vi "Periodic Tasks.vi"(8 "error in":errorcluster) -> ()   [LabVIEW 2014]
doc: "This VI runs in parallel to other tasks. It can contain as many user-defined periodic loops as you need. These can carry out PID or other sorts of timed response."
uses:
  <vilib>/Rock Robotics/WPI/Solenoid/WPI_SolenoidValue.ctl
  <vilib>/Rock Robotics/WPI/Joystick/WPI_JoystickGetSetRefNum.vi
  <vilib>/Rock Robotics/WPI/RobotDrive/WPI_RobotDriveGetSetRefNum.vi
  Robot Global Data.vi
  <vilib>/Rock Robotics/WPI/Solenoid/WPI_SolenoidSetEnum.vi
panel:
  out "Encoder (INCH)":dbl format="%#_10g"
  in  "error in 2":errorcluster
  in  "X-Slew Rate":dbl=0.05
  in  "Y-Slew Rate":dbl=0.05
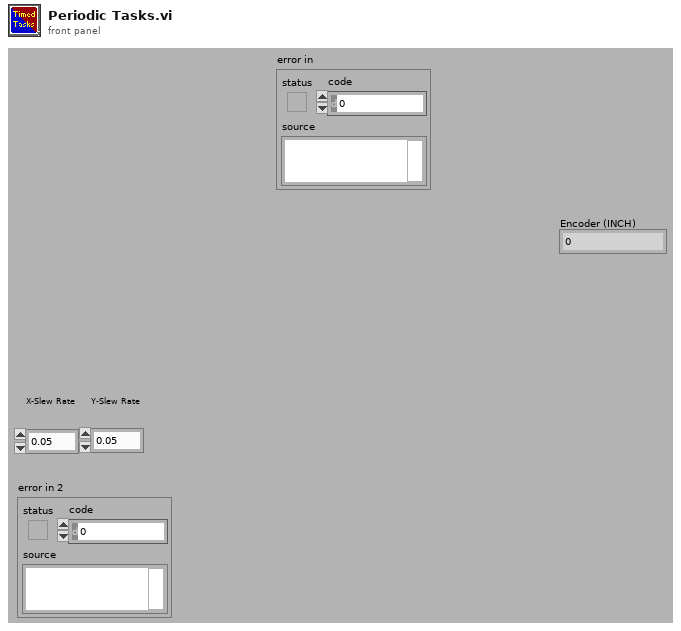
[diagram p1: front panel]
types:
  T1 = typedef "WPI_EncoderDevRef.ctl" = cluster{"DevStatus":errorcluster, "EncoderIndex":T2, "CounterIndex":T3, "DistancePerCount":dbl, "Decoding Type":T4}
  T2 = typedef "FPGA_EncoderIdx.ctl" = enum8{"Enc 0", "Enc 1", "Enc 2", "Enc 3", "Enc 4", "Enc 5", "Enc 6", "Enc 7", "Invalid"}
  T3 = typedef "FPGA_CounterCtrSystemIndex.ctl" = enum8{"Ctr 0", "Ctr 1", "Ctr 2", "Ctr 3", "Ctr 4", "Ctr 5", "Ctr 6", "Ctr 7", "Invalid"}
  T4 = typedef "WPI_EncoderType.ctl" = enum16{"1x", "2x", "4x"}
  T5 = typedef "WPI_RobotDriveDevRef.ctl" = cluster{"DevStatus":errorcluster, "Motors[]":T6[], "Square Inputs":bool, "Max Output":dbl}
  T6 = typedef "WPI_MotorControlDeviceRef.ctl" = cluster{"DeviceStatus":errorcluster, "Type":T7, "PWM":cluster{"Controller":T8, "PWM Channel":T9, "DeadBand":T10}, "CAN":cluster{"Device Number":u8, "Control Mode":T11, "Semaphore":T12, "Max Vout":dbl, "TalonSRX Control Mode":T13}, "Invert":bool, "TransformRef":T14, "InvTransformRef":T14}
  T7 = typedef "WPI_MotorControlType.ctl" = enum16{"PWM", "CAN", "CANTalonSRX"}
  T8 = typedef "FPGA_TypedefDigitalModule.ctl" = enum16{"Controller 1"}
  T9 = typedef "FPGA_DIOPWMChannel.ctl" = enum8{"PWM 0", "PWM 1", "PWM 2", "PWM 3", "PWM 4", "PWM 5", "PWM 6", "PWM 7", "PWM 8", "PWM 9", "PWM MXP 0", "PWM MXP 1", "PWM MXP 2", "PWM MXP 3", "PWM MXP 4", "PWM MXP 5", "PWM MXP 6", "PWM MXP 7", "PWM MXP 8", "PWM MXP 9", "Invalid"}
  T10 = typedef "WPI_PWMDeadband.ctl" = cluster{"Name":string, "maxPositivePwm":i32, "minPositivePwm":i32, "centerPwm":i32, "maxNegativePwm":i32, "minNegativePwm":i32, "angularRange":u16}
  T11 = typedef "WPI_CANJaguar_ControlMode.ctl" = enum8{"Percent VBus", "Current", "Speed", "Position", "Voltage"}
  T12 = typedef "Semaphore RefNum" = refnum<k1>
  T13 = typedef "WPI_CANTalonSRX_APIControlMode.ctl" = enum8{"Percent VBus", "Speed", "Position", "Slave", "Unchanged / Invalid"}
  T14 = typedef "WPI_PWMTransform_ConPane.ctl" = refnum<vi>
  T15 = typedef "WPI_JoystickDevRef.ctl" = cluster{"Device":T16}
  T16 = typedef "WPI_JoystickDeviceEnum.ctl" = enum16{"USB 0", "USB 1", "USB 2", "USB 3", "USB 4", "USB 5"}
  T17 = cluster{"JoystickDevRef":T15, "RobotDriveDevRef":T5}
  T18 = typedef "WPI_SolenoidDevRef.ctl" = cluster{"DevStatus":errorcluster, "Pneumatics Control Module":u8, "Forward Solenoid Channel":T19, "Reverse Solenoid Channel":T19}
  T19 = typedef "WPI_SolenoidChannel.ctl" = enum8{"Solenoid 0", "Solenoid 1", "Solenoid 2", "Solenoid 3", "Solenoid 4", "Solenoid 5", "Solenoid 6", "Solenoid 7", "Invalid"}
  T20 = typedef "WPI_SolenoidValue.ctl" = enum16{"Off", "On", "Forward", "Reverse"}
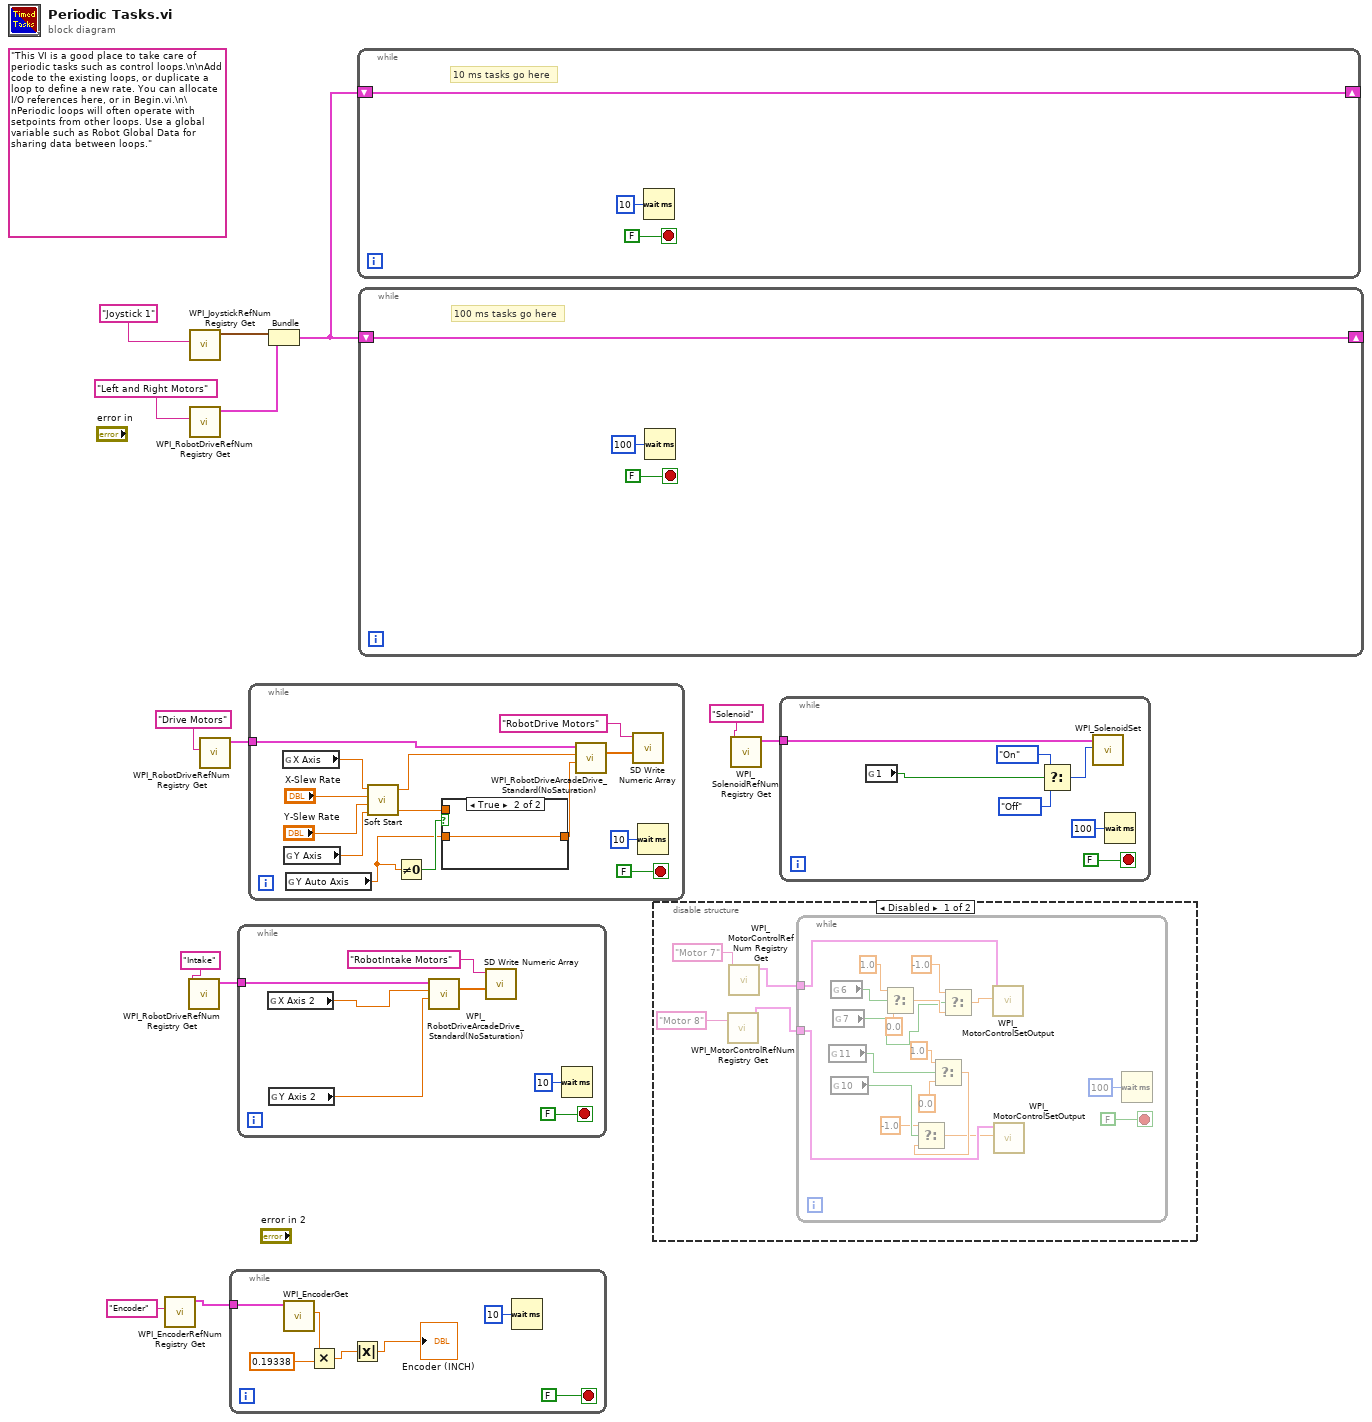
[diagram p0: block diagram]
diagram:
  (unwired) "This VI is a good place to take care of periodic tasks such as control loops.\n\nAdd code to the existing loops, or duplicate a loop to define a new rate. You can allocate I/O references here, or in Begin.vi.\n\nPeriodic loops will often operate with setpoints from other loops. Use a global variable such as Robot Global Data for sharing data between loops."
  n1 = call <vilib>:"WPI_EncoderRefNum Registry Get.vi"("refnum name"="Encoder") -> ("EncoderDevRef"=w1:T1)  [unwired: 9 in, 1 out]
  n2 = call <vilib>:"WPI_RobotDriveRefNum Registry Get.vi"("refnum name"="Intake") -> ("RobotDriveDevRef"=w3:T5)  [unwired: 1 in, 9 out]
  n3 = call <vilib>:"WPI_JoystickRefNum Registry Get.vi"("refnum name"="Joystick 1") -> ("JoystickDevRef"=w11:T15)  [unwired: 1 in, 9 out]
  n4 = call <vilib>:"WPI_RobotDriveRefNum Registry Get.vi"("refnum name"="Left and Right Motors") -> ("RobotDriveDevRef"=w10:T5)  [unwired: 1 in, 9 out]
  n5 = call <vilib>:"WPI_RobotDriveRefNum Registry Get.vi"("refnum name"="Drive Motors") -> ("RobotDriveDevRef"=w7:T5)  [unwired: 1 in, 9 out]
  n6 = while {
    tunnel: w1 -> [w19]
    stop <- FALSE stop-if-true
    n7 = call <vilib>:"WPI_EncoderGet.vi"("EncoderDevRef"=w19) -> ("Distance"=w18:dbl)  [unwired: 5 in, 5 out]
    n8 = Multiply(x=w18, y=0.19338 ("x")) -> (x*y=w15:dbl)
    n9 = Absolute Value(x=w15) -> (abs(x)=→"Encoder (INCH)":dbl)
    n10 = Wait (ms)(milliseconds to wait=u32 10) -> ()  [unwired: 1 out]
  }
  n11 = while {
    tunnel: w3 -> [w23]
    stop <- FALSE stop-if-true
    n12 = global read "Robot Global Data.vi" "X Axis 2"() -> (w21:dbl)
    n13 = global read "Robot Global Data.vi" "Y Axis 2"() -> (w22:dbl)
    n14 = call <vilib>:"WPI_RobotDriveArcadeDrive_Standard(NoSaturation).vi"("Y axis value"=w22, "X axis value"=w21, "RobotDriveDevRef"=w23) -> ("Motor Values"=w24:dbl[])  [unwired: 1 in, 7 out]
    n15 = call <vilib>:"SD Write Numeric Array.vi"("Numeric Array"=w24, "Name"="RobotIntake Motors") -> ()  [unwired: 8 in, 2 out]
    n16 = Wait (ms)(milliseconds to wait=u32 10) -> ()  [unwired: 1 out]
  }
  n17 = while {
    tunnel: w7 -> [w37]
    stop <- FALSE stop-if-true
    n18 = global read "Robot Global Data.vi" "X Axis"() -> (w36:dbl)
    n19 = global read "Robot Global Data.vi" "Y Axis"() -> (w35:dbl)
    n20 = global read "Robot Global Data.vi" "Y Auto Axis"() -> (w28:dbl)
    n21 = call "Soft Start.vi"("Y-axis Joystick"=w35, "Y-Slew Rate"="Y-Slew Rate", "X-Slew Rate"="X-Slew Rate", "X- axis Joystick"=w36) -> ("Y-axis drive"=w29:dbl, "X-axis drive"=w34:dbl)  [unwired: 1 in]
    n22 = Not Equal To 0?(x=w28) -> (x != 0?=w31:bool)
    n23 = case shown="True" w31 {
      tunnel: [w42 w43] -> w30
      tunnel: w28 -> [_ w43]
      tunnel: w29 -> [w42 _]
      frame False {
      }
      frame True {
      }
    }
    n24 = call <vilib>:"WPI_RobotDriveArcadeDrive_Standard(NoSaturation).vi"("Y axis value"=w30, "X axis value"=w34, "RobotDriveDevRef"=w37) -> ("Motor Values"=w38:dbl[])  [unwired: 1 in, 7 out]
    n25 = call <vilib>:"SD Write Numeric Array.vi"("Numeric Array"=w38, "Name"="RobotDrive Motors") -> ()  [unwired: 8 in, 2 out]
    n26 = Wait (ms)(milliseconds to wait=u32 10) -> ()  [unwired: 1 out]
  }
  n27 = Bundle("JoystickDevRef"=w11, "RobotDriveDevRef"=w10) -> (w9:T17)  [unwired: 1 out]
  n28 = while {
    shift-right: [w44] -> _
    shift-left: w9 -> [w44]
    stop <- FALSE stop-if-true
    # "10 ms tasks go here"
    n29 = Wait (ms)(milliseconds to wait=u32 10) -> ()  [unwired: 1 out]
  }
  n30 = while {
    shift-right: [w47] -> _
    shift-left: w9 -> [w47]
    stop <- FALSE stop-if-true
    # "100 ms tasks go here"
    n31 = Wait (ms)(milliseconds to wait=u32 100) -> ()  [unwired: 1 out]
  }
  n32 = disable-structure shown="Disabled" {
    frame Disabled {
      n33 = call <vilib>:"WPI_MotorControlRefNum Registry Get.vi"("refnum name"="Motor 8") -> ("MotorControlDevRef"=w50:T6)  [unwired: 9 in, 1 out]
      n34 = call <vilib>:"WPI_MotorControlRefNum Registry Get.vi"("refnum name"="Motor 7") -> ("MotorControlDevRef"=w51:T6)  [unwired: 9 in, 1 out]
      n35 = while {
        tunnel: w51 -> [w69]
        tunnel: w50 -> [w68]
        stop <- FALSE stop-if-true
        n36 = global read "Robot Global Data.vi" "11"() -> (w66:bool)
        n37 = global read "Robot Global Data.vi" "6"() -> (w58:bool)
        n38 = global read "Robot Global Data.vi" "10"() -> (w64:bool)
        n39 = global read "Robot Global Data.vi" "7"() -> (w57:bool)
        n40 = Select(t=1.0, s=w58, f=0.0) -> (s? t:f=w62:dbl)
        n41 = Select(t=1.0, s=w66, f=0.0) -> (s? t:f=w56:dbl)
        n42 = Select(t=-1.0, s=w64, f=w56) -> (s? t:f=w55:dbl)
        n43 = Select(t=-1.0, s=w57, f=w62) -> (s? t:f=w54:dbl)
        n44 = call <vilib>:"WPI_MotorControlSetOutput.vi"("Output"=w54, "MotorControlDevRef"=w69) -> ()  [unwired: 7 in, 3 out]
        n45 = call <vilib>:"WPI_MotorControlSetOutput.vi"("Output"=w55, "MotorControlDevRef"=w68) -> ()  [unwired: 7 in, 3 out]
        n46 = Wait (ms)(milliseconds to wait=u32 100) -> ()  [unwired: 1 out]
      }
    }
    frame Enabled {
    }
  }
  n47 = call <vilib>:"WPI_SolenoidRefNum Registry Get.vi"("refnum name"="Solenoid") -> ("SolenoidDevRef"=w5:T18)  [unwired: 9 in, 1 out]
  n48 = while {
    tunnel: w5 -> [w73]
    stop <- FALSE stop-if-true
    n49 = global read "Robot Global Data.vi" "1"() -> (w72:bool)
    n50 = Select(t=WPI_SolenoidValue."On" ("Value"), s=w72, f=WPI_SolenoidValue."Off" ("Value")) -> (s? t:f=w74:T20)
    n51 = call-poly <vilib>:"WPI_SolenoidSet.vi"("Value"=w74, "SolenoidDevRef"=w73) -> ()  [unwired: 8 in, 2 out]
    n52 = Wait (ms)(milliseconds to wait=u32 100) -> ()  [unwired: 1 out]
  }
